vi "整理批次号-时间-结果-数据.vi"(11 "存档数据和结果":T1) -> (0 "添加了批次号时间，结果的存档颜色":bool[](array[boolean]), 3 "数组":string[](array[string]))   [LabVIEW 2014]
uses:
  Global.vi
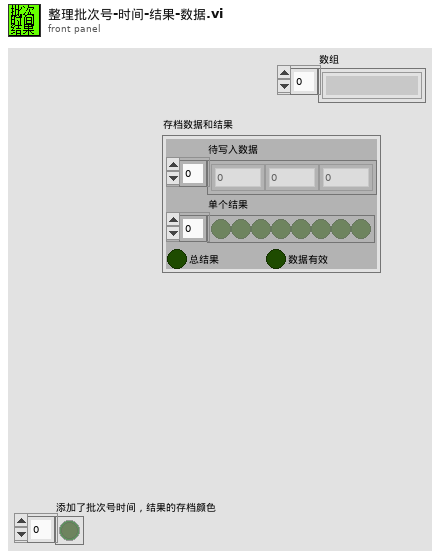
[diagram p1: front panel]
types:
  T1 = typedef "存档数据和结果.ctl" = cluster{"待写入数据":dbl[], "单个结果":bool[], "总结果":bool, "数据有效":bool}
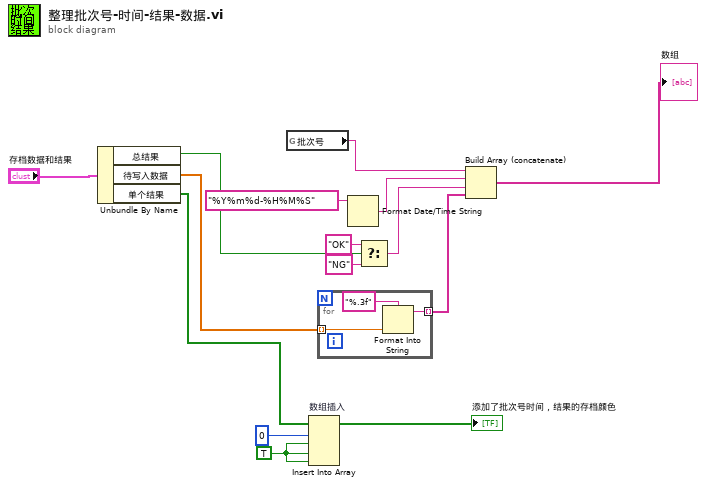
[diagram p0: block diagram]
diagram:
  w2 = TRUE ("新元素/子数组")
  n1 = Unbundle By Name("存档数据和结果") -> ("总结果"=w8:bool, "待写入数据"=w7:dbl[], "单个结果"=w4:bool[])
  n2 = global read "Global.vi" "批次号"() -> (w1:string)
  n3 = Insert Into Array "数组插入"(array=w4, index=0 ("索引"), new element #1=w2, new element #2=w2, new element #3=w2) -> (→"添加了批次号时间，结果的存档颜色":bool[])
  n4 = for {
    tunnel: w7 -> [w18] mode=indexing
    tunnel: [w17] -> w6 mode=indexing
    n5 = Format Into String(format string="%.3f" ("格式字符串"), w18) -> (resulting string=w17:string)  [unwired: 2 in, 1 out]
  }
  n6 = Format Date/Time String(time format string (%c)="%Y%m%d-%H%M%S") -> (date/time string=w15:string)  [unwired: 2 in]
  n7 = Select(t="OK", s=w8, f="NG") -> (s? t:f=w12:string)
  n8 = Build Array (concatenate)(w1, w15, w12, w6) -> (→"数组":string[])
